vi "phase corrector.vi"(1 "Phase":dbl) -> (0 "Corrected phase":dbl)   [LabVIEW 2021]
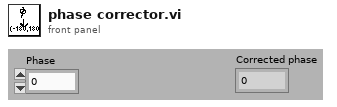
[diagram p1: front panel]
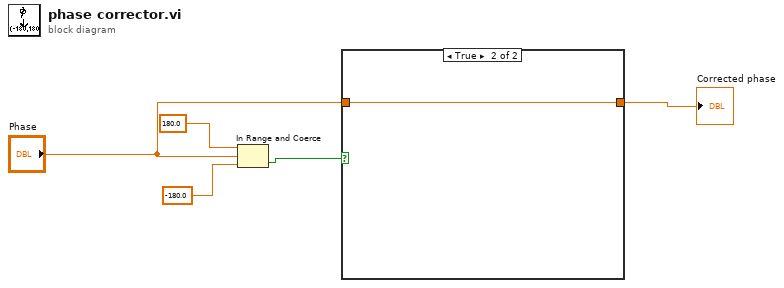
[diagram p0: block diagram]
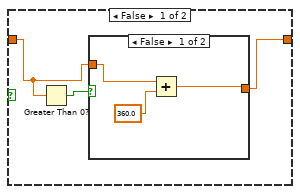
[diagram p2: hidden frame]
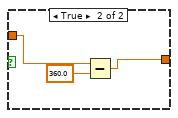
[diagram p3: hidden frame]
diagram:
  n1 = In Range and Coerce(upper limit=180.0, x="Phase", lower limit=-180.0) -> (In Range?=w3:bool)  [unwired: 1 out]
  n2 = case shown="True" w3 {
    tunnel: "Phase" -> [w6 w15]
    tunnel: [w7 w15] -> w1
    frame False {
      n3 = Greater Than 0?(x=w6) -> (x > 0?=w8:bool)
      n4 = case shown="False" w8 {
        tunnel: w6 -> [w11 w14]
        tunnel: [w9 w12] -> w7
        frame False {
          n5 = Add(x=w11, y=360.0) -> (x+y=w9:dbl)
        }
        frame True {
          n6 = Subtract(x=w14, y=360.0) -> (x-y=w12:dbl)
        }
      }
    }
    frame True {
    }
  }
  "Corrected phase" <- w1
